vi "Close Excel File.vi"(8 "Error In":errorcluster, 11 "ExcelRefs":T1) -> (0 "Error Out":errorcluster)   [LabVIEW 2011]
uses:
  Controls/Excel Refs.ctl
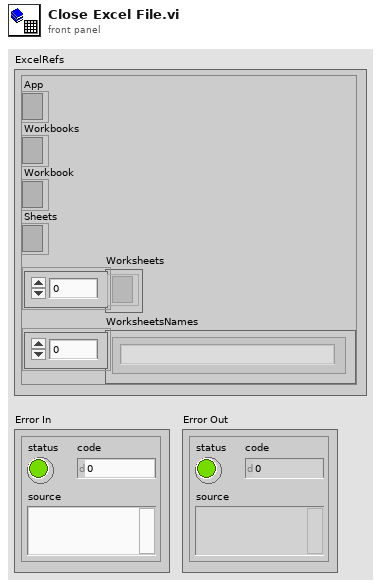
[diagram p1: front panel]
types:
  T1 = typedef "Excel Refs.ctl" = cluster{"App":refnum<k7>, "Workbooks":refnum<k7>, "Workbook":refnum<k7>, "Sheets":refnum<k7>, "Worksheets":refnum<k7>[], "WorksheetsNames":string[]}
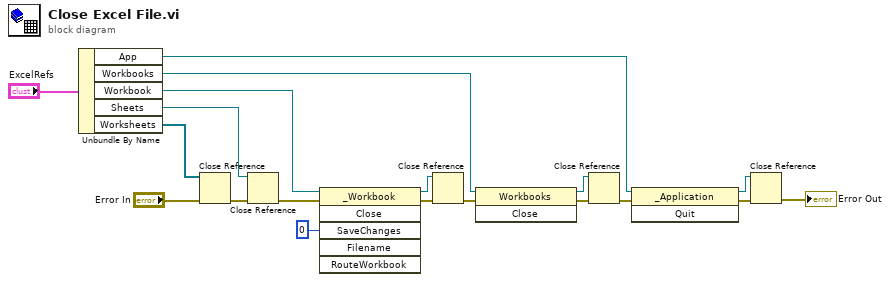
[diagram p0: block diagram]
diagram:
  n1 = Unbundle By Name("ExcelRefs") -> ("App"=w2:refnum<k7>, "Workbooks"=w3:refnum<k7>, "Workbook"=w4:refnum<k7>, "Sheets"=w15:refnum<k7>, "Worksheets"=w17:refnum<k7>[])
  n2 = Close Reference(reference=w17, error in (no error)="Error In") -> (error out=w16:errorcluster)
  n3 = Close Reference(reference=w15, error in (no error)=w16) -> (error out=w5:errorcluster)
  n4 = invoke class="_Workbook" method="Close"(reference=w4, error in=w5, "SaveChanges"=0) -> (reference out=w7:refnum<k7>, error out=w6:errorcluster)  [unwired: 3 in, 4 out]
  n5 = Close Reference(reference=w7, error in (no error)=w6) -> (error out=w8:errorcluster)
  n6 = invoke class="Workbooks" method="Close"(reference=w3, error in=w8) -> (reference out=w10:refnum<k7>, error out=w9:errorcluster)  [unwired: 1 in, 1 out]
  n7 = Close Reference(reference=w10, error in (no error)=w9) -> (error out=w13:errorcluster)
  n8 = invoke class="_Application" method="Quit"(reference=w2, error in=w13) -> (reference out=w11:refnum<k7>, error out=w12:errorcluster)  [unwired: 1 in, 1 out]
  n9 = Close Reference(reference=w11, error in (no error)=w12) -> (error out=→"Error Out":errorcluster)
